vi "Formate Assertions for Description.vi"(10 "Item":string, 11 "Result Model In":refnum<class "Result Model.lvclass">) -> (2 "Assertions Description":string)   [LabVIEW 2020, in "Result Model.lvclass"]
uses:
  Result Model.lvclass
  Result Model.lvclass/Result Model.ctl
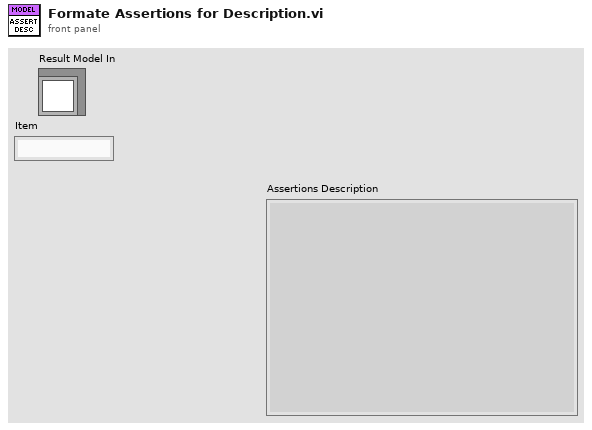
[diagram p1: front panel]
types:
  T1 = typedef "Result.lvlib/Type.ctl" = enum16{"Test Case", "Test Suite", "Test Run", "Pass", "Fail", "Skip", "Pass if", "Fail if", "Pass if Error", "Fail if Error", "Pass if Equal", "Fail if Equal"}
  T2 = typedef "Result.lvlib/Status.ctl" = enum16{"", "Passed", "Failed", "Error", "Skipped", "Setup Error", "Broken", "Teardown Error"}
  T3 = map{string, cluster{"Result Type":T1, "Status":T2, "Description":string, "Data":cluster{"Expected":variant, "Actual":variant, "Delta":variant}}[]}
  T4 = cluster{"Result Type":T1, "Status":T2, "Description":string, "Data":cluster{"Expected":variant, "Actual":variant, "Delta":variant}}[]
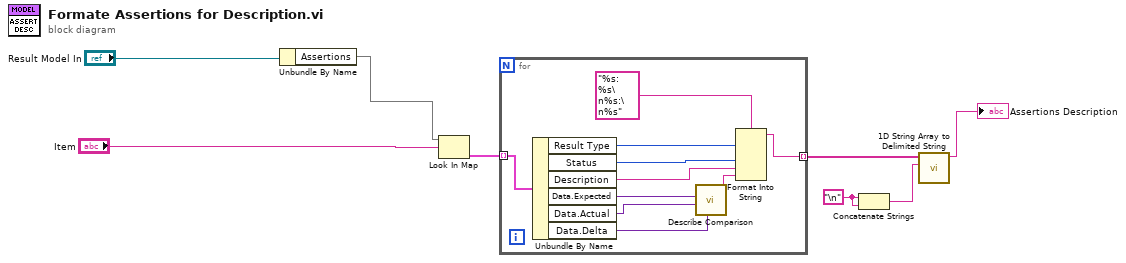
[diagram p0: block diagram]
diagram:
  w3 = "\n"
  n1 = Unbundle By Name("Result Model In") -> ("Assertions"=w1:T3)
  n2 = Look In Map(map=w1, key="Item") -> (value=w5:T4)  [unwired: 1 in, 1 out]
  n3 = for {
    tunnel: [w17] -> w8 mode=indexing
    tunnel: w5 -> [w14] mode=indexing
    n4 = Unbundle By Name(w14) -> ("Result Type"=w16:T1, "Status"=w15:T2, "Description"=w13:string, "Data.Expected"=w11:variant, "Data.Actual"=w10:variant, "Data.Delta"=w9:variant)
    n5 = call "Describe Comparison.vi"("Delta"=w9, "Actual"=w10, "Expected"=w11) -> ("Description"=w12:string)  [unwired: 8 in]
    n6 = Format Into String(format string="%s: %s\n%s:\n%s", w16, w15, w13, w12) -> (resulting string=w17:string)  [unwired: 2 in, 1 out]
  }
  n7 = Concatenate Strings(w3, w3) -> (w4:string)
  n8 = call <vilib>:"1D String Array to Delimited String.vi"("delimiter"=w4, "string array"=w8) -> ("delimited string"=→"Assertions Description":string)  [unwired: 9 in]
